vi "ToHotGoalType.vi"(11 "IntIn":i32) -> (3 "EnumOut":T1)   [LabVIEW 2013]
uses:
  HotGoalDetectType.ctl
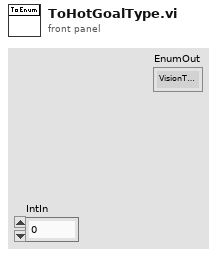
[diagram p1: front panel]
types:
  T1 = typedef "HotGoalDetectType.ctl" = enum16{"VisionTarget", "Kinect"}
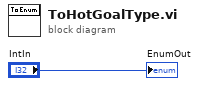
[diagram p0: block diagram]
diagram:
  "EnumOut" <- "IntIn"
